vi "Stop All Event.vi"(8 "error in":errorcluster) -> (0 "error out":errorcluster)   [LabVIEW 2014, in "Events Lib.lvlib"]
uses:
  Events Lib.lvlib
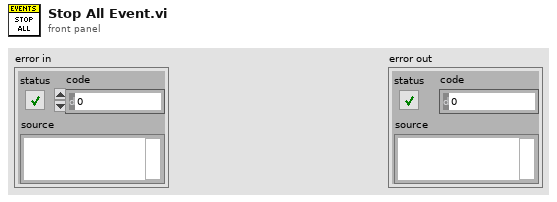
[diagram p1: front panel]
types:
  T1 = typedef "Events Lib.lvlib/Events TypeDef.ctl" = cluster{"Stop Event":refnum<user-event>}
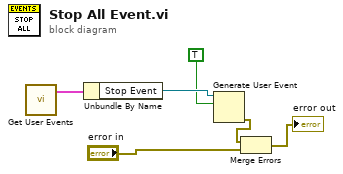
[diagram p0: block diagram]
diagram:
  n1 = call "Get User Events.vi"() -> ("User Events Ref"=w6:T1)  [unwired: 10 in, 1 out]
  n2 = Unbundle By Name(w6) -> ("Stop Event"=w5:refnum<user-event>)
  n3 = Generate User Event(user event=w5, event data cluster=TRUE) -> (error out=w3:errorcluster)  [unwired: 2 in, 1 out]
  n4 = Merge Errors(w3, "error in") -> (→"error out":errorcluster)
